vi "ExecuteCommand.vi"(6 "return immediately":bool, 8 "error in (no error)":errorcluster, 10 "code":string, 11 "controller in":refnum<k24>) -> (0 "error out":errorcluster, 2 "return value":string, 3 "controller out":refnum<k24>)   [LabVIEW 2019]
uses:
  C:/Users/patrick/Documents/GitHub/Aerotech-Delay-Line/lvsrc/Aerotech-Ensemble-LabVIEW/2010-5.6/Bin/Aerotech.Ensemble.dll
  Bin/Aerotech.Ensemble.dll
panel:
  in  "Null 2":refnum<k24>
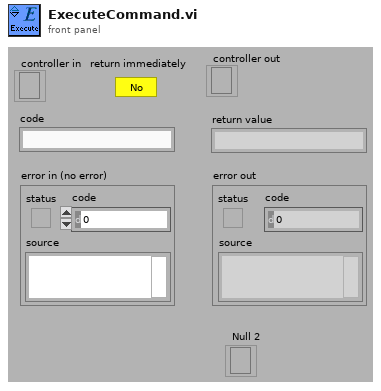
[diagram p1: front panel]
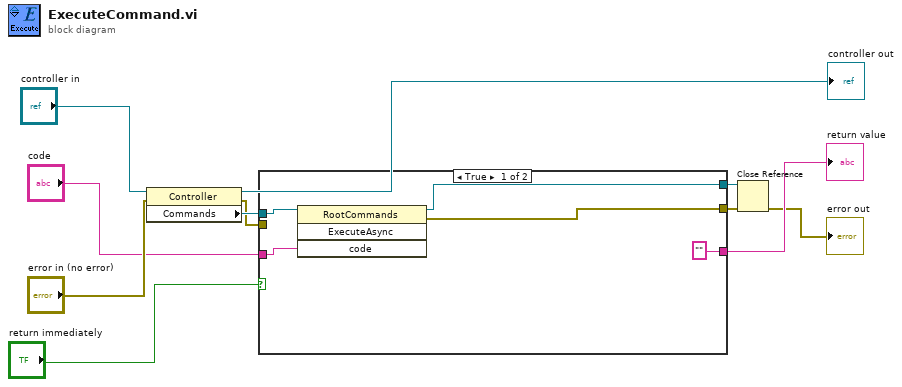
[diagram p0: block diagram]
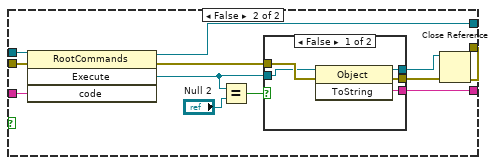
[diagram p2: hidden frame]
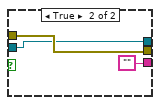
[diagram p3: hidden frame]
diagram:
  n1 = property class="Controller"(reference="controller in", error in="error in (no error)") -> (reference out=→"controller out":refnum<k24>, error out=w5:errorcluster, "Commands"=w6:refnum<k24>)
  n2 = case shown="True" "return immediately" {
    tunnel: "code" -> [w13 w28]
    tunnel: ["" w26] -> w7
    tunnel: w6 -> [w16 w22]
    tunnel: w5 -> [_ w21]
    tunnel: [w14 w20] -> w4
    tunnel: [w15 w17] -> w2
    frame True {
      n3 = invoke class="RootCommands" method="ExecuteAsync"(reference=w16, "code"=w13) -> (reference out=w15:refnum<k24>, error out=w14:errorcluster)  [unwired: 2 in, 2 out]
    }
    frame False {
      n4 = invoke class="RootCommands" method="Execute"(reference=w22, error in=w21, "code"=w28) -> (reference out=w17:refnum<k24>, error out=w27:errorcluster, "Execute"=w24:refnum<k24>)  [unwired: 1 in, 1 out]
      n5 = Equal?(x=w24, y="Null 2") -> (x = y?=w25:bool)
      n6 = case shown="False" w25 {
        tunnel: w27 -> [w33 w36]
        tunnel: [w32 w36] -> w19
        tunnel: w24 -> [w31 w34]
        tunnel: [w30 ""] -> w26
        tunnel: [w29 w34] -> w18
        frame False {
          n7 = invoke class="Object" method="ToString"(reference=w31, error in=w33) -> (reference out=w29:refnum<k24>, error out=w32:errorcluster, "ToString"=w30:string)  [unwired: 1 in]
        }
        frame True {
        }
      }
      n8 = Close Reference(reference=w18, error in (no error)=w19) -> (error out=w20:errorcluster)
    }
  }
  "return value" <- w7
  n9 = Close Reference(reference=w2, error in (no error)=w4) -> (error out=→"error out":errorcluster)
